vi "Motor polarity mMc.vi"(0 "Mot pol in":bool caption="Motor polarity in", 1 "Port":T1={"P type"=0, "reference"="", " Terminator "="\r\n", "Timeout"=300} {"Timeout" step=10; "P type" items=["none", "RS-232C"]}, 3 "error in (no error)":errorcluster, 4 "set/get":bool caption="set\n\n\nget", 5 "Controller #":string) -> (6 "Mot pol out":bool caption="Motor polarity out", 9 "error out":errorcluster)   [LabVIEW 2011]
panel:
  # "Motor polarity"
  # "open      closed"
  # "open      closed"
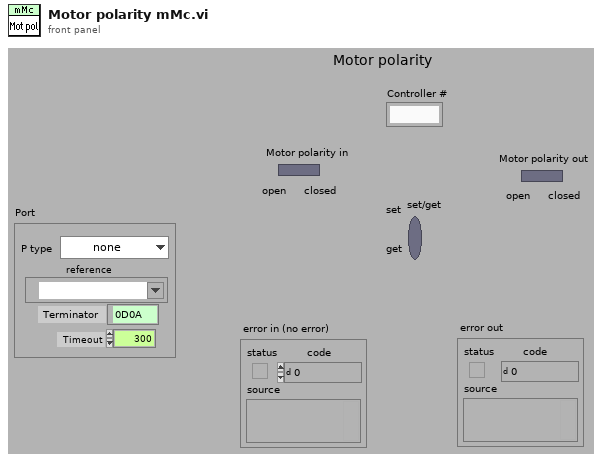
[diagram p1: front panel]
types:
  T1 = cluster{"P type":u16, "reference":refnum<visa-resource-name>, " Terminator ":string, "Timeout":i32}
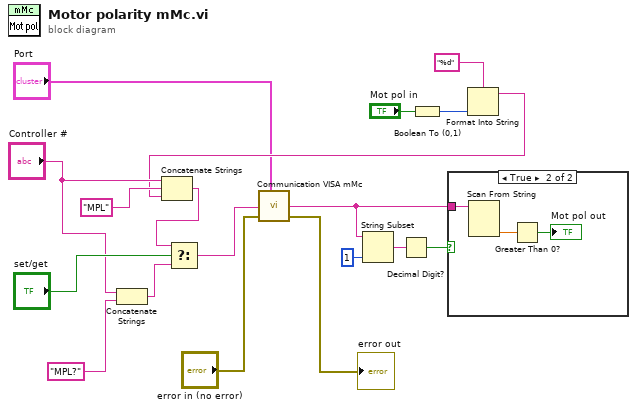
[diagram p0: block diagram]
diagram:
  n1 = Concatenate Strings("Controller #", "MPL?") -> (w18:string)
  n2 = Boolean To (0,1)(Boolean="Mot pol in") -> (0, 1=w6:i16)
  n3 = Format Into String(format string="%d", w6) -> (resulting string=w8:string)  [unwired: 2 in, 1 out]
  n4 = Concatenate Strings("Controller #", "MPL", w8) -> (w16:string)
  n5 = Select(t=w16, s="set/get", f=w18) -> (s? t:f=w15:string)
  n6 = call "Communication VISA mMc.vi"("Port"="Port", "Command"=w15, "error in (no error)"="error in (no error)") -> ("Return"=w1:string, "error out"=→"error out":errorcluster)  [unwired: 3 in, 2 out]
  n7 = String Subset(string=w1, length (rest)=1 ("length (rest)")) -> (substring=w3:string)  [unwired: 1 in]
  n8 = Decimal Digit?(1:w3) -> (0:w2:bool)
  n9 = case shown="True" w2 {
    tunnel: w1 -> [_ w21]
    frame False {
    }
    frame True {
      n10 = Scan From String(input string=w21) -> (output 1=w20:dbl)  [unwired: 4 in, 3 out]
      n11 = Greater Than 0?(x=w20) -> (x > 0?=→"Mot pol out":bool)
    }
  }
